vi "Setting_2.vi"() -> ()   [LabVIEW 2015]
uses:
  0.Control/Setting_Control_Main_Inspection_Item Action.ctl
  0.Control/Setting_Control_Main Action.ctl
  <vilib>/vision/Measure.llb/Edge Options.ctl
  <vilib>/vision/Measure.llb/Edge Polarity.ctl
  <vilib>/vision/Measure.llb/Straight Edge Options.ctl
  <vilib>/vision/Measure.llb/Straight Edge Process.ctl
  <vilib>/Utility/miscctls.llb/LVPointTypeDef.ctl
  0.Control/Setting_Control_Pattern Paremeter.ctl
  <vilib>/userdefined/High Color/IMAQdx.ctl
  <vilib>/vision/NI_Vision_Development_Module.lvlib
panel:
  in  "ROIsize":cluster{"Width":dbl, "Height":dbl}[](array[cluster])=[{"Width"=0.375, "Height"=0.2}, {"Width"=0.375, "Height"=0.2}, {"Width"=0.375, "Height"=0.2}, {"Width"=0.375, "Height"=0.2}]
  in  "Don't need to press Ctrl To ZoomIn/ZoomOut":bool
  in  "ROI數量":i32=4
  in  "檢測項目":T1
  in  "確認檢測項目":bool
  in  "Tab Control":enum32{"設定", "тX把计", "тY把计", "補正參數"}(tab)
  in  "單步測試":bool
  in  "連續測試":bool
  in  "取像":bool
  in  "連續取像":bool
  in  "離開":bool
  in  "匯入圖片":bool
  out "Coordinate System":T2 {"Measurement System"."Axis Reference" items=["Direct", "Indirect"]; "Measurement System"."Angle (deg)" format="%.2f"; "Measurement System"."Origin"."Y" format="%.2f"; "Measurement System"."Origin"."X" format="%.2f"; "Reference System"."Axis Reference" items=["Direct", "Indirect"]; "Reference System"."Angle (deg)" format="%.2f"; "Reference System"."Origin"."Y" format="%.2f"; "Reference System"."Origin"."X" format="%.2f"}
  in  "start path":path=path "D:/渦輪組裝機參數/Data 資料/Setting Data"
  in  "file (use dialog)":path=path "D:/渦輪組裝機參數/Data 資料/Setting Data"
  out "Main Axis 2":T3 {"Point2"."Y" format="%.2f"; "Point2"."X" format="%.2f"; "Point1"."Y" format="%.2f"; "Point1"."X" format="%.2f"}
  out "Secondary Axis 2":T3 {"Point2"."Y" format="%.2f"; "Point2"."X" format="%.2f"; "Point1"."Y" format="%.2f"; "Point1"."X" format="%.2f"}
  out "Main Axis":T3 {"Point2"."Y" format="%.2f"; "Point2"."X" format="%.2f"; "Point1"."Y" format="%.2f"; "Point1"."X" format="%.2f"}
  out "Secondary Axis":T3 {"Point2"."Y" format="%.2f"; "Point2"."X" format="%.2f"; "Point1"."Y" format="%.2f"; "Point1"."X" format="%.2f"}
  in  "Direction":u16(ring)
  in  "LayoutOptions":T4={"Show Search Area"=FALSE, "Show Search Lines"=FALSE, "Show Edges Found"=FALSE, "Show Result"=TRUE, "Search Area Color"=65280, "Search Lines Color"=255, "Edge Locations Color"=16776960, "Result Color"=16711680, "Overlay Group Name"=""}
  in  "Primary Line Fit Options":T5={"Number of Lines"=1, "Type"=enum."First Edge Rake", "Min. Score"=10.0, "Max. Score"=1000.0, "Orientation"=0.0, "Angle Range"=45.0, "Angle Tolerance"=1.0, "Step Size"=7, "Min. SNR (db)"=0.0, "Min. Points (%)"=25.0, "Hough Iterations"=5} {"Min. Points (%)" min=0.0 max=100.0; "Min. SNR (db)" min=0.0; "Max. Score" min=0.0 max=1024.0; "Min. Score" min=0.0 max=1024.0 step=1.0}
  in  "Secondary Line Fit Options":T5={"Number of Lines"=1, "Type"=enum."First Edge Rake", "Min. Score"=10.0, "Max. Score"=1000.0, "Orientation"=0.0, "Angle Range"=45.0, "Angle Tolerance"=1.0, "Step Size"=7, "Min. SNR (db)"=0.0, "Min. Points (%)"=25.0, "Hough Iterations"=5} {"Min. Points (%)" min=0.0 max=100.0; "Min. SNR (db)" min=0.0; "Max. Score" min=0.0 max=1024.0; "Min. Score" min=0.0 max=1024.0 step=1.0}
  in  "Options":T9={"Direction"=0, "Primary Edge Options"={"Edge Polarity"=0, "Kernel Size"=3, "Width"=3, "Minimum Edge Strength"=10.0, "Interpolation Type"=enum."Bilinear Fixed", "Data Processing Method"=enum."Average"}, "Secondary Edge Options"={"Edge Polarity"=0, "Kernel Size"=3, "Width"=3, "Minimum Edge Strength"=10.0, "Interpolation Type"=enum."Bilinear Fixed", "Data Processing Method"=enum."Average"}, "Show Search Area"=FALSE, "Show Search Lines"=FALSE, "Show Edges Found"=FALSE, "Show Result"=TRUE, "Search Area Color"=65280, "Search Lines Color"=255, "Edge Locations Color"=16776960, "Result Color"=16711680, "Overlay Group Name"=""} {"Secondary Edge Options"."Edge Polarity" items=["All Edges", "Rising Edges", "Falling Edges"]; "Secondary Edge Options"."Minimum Edge Strength" format="%.2f"; "Secondary Edge Options"."Width" step=2; "Secondary Edge Options"."Kernel Size" step=2; "Primary Edge Options"."Edge Polarity" items=["All Edges", "Rising Edges", "Falling Edges"]; "Primary Edge Options"."Minimum Edge Strength" format="%.2f"; "Primary Edge Options"."Width" step=2; "Primary Edge Options"."Kernel Size" step=2}
  out "Image":T10(plugin-control)
  out "Pattern":T10(plugin-control)
  out "Set action":T11
  in  "相機、光源":T12 {"光源亮度" step=1 scale=0.0..255.0; "相機選擇" items=["相機 1", "相機 2"]; "光源選擇" items=["光源 1", "光源 2"]}
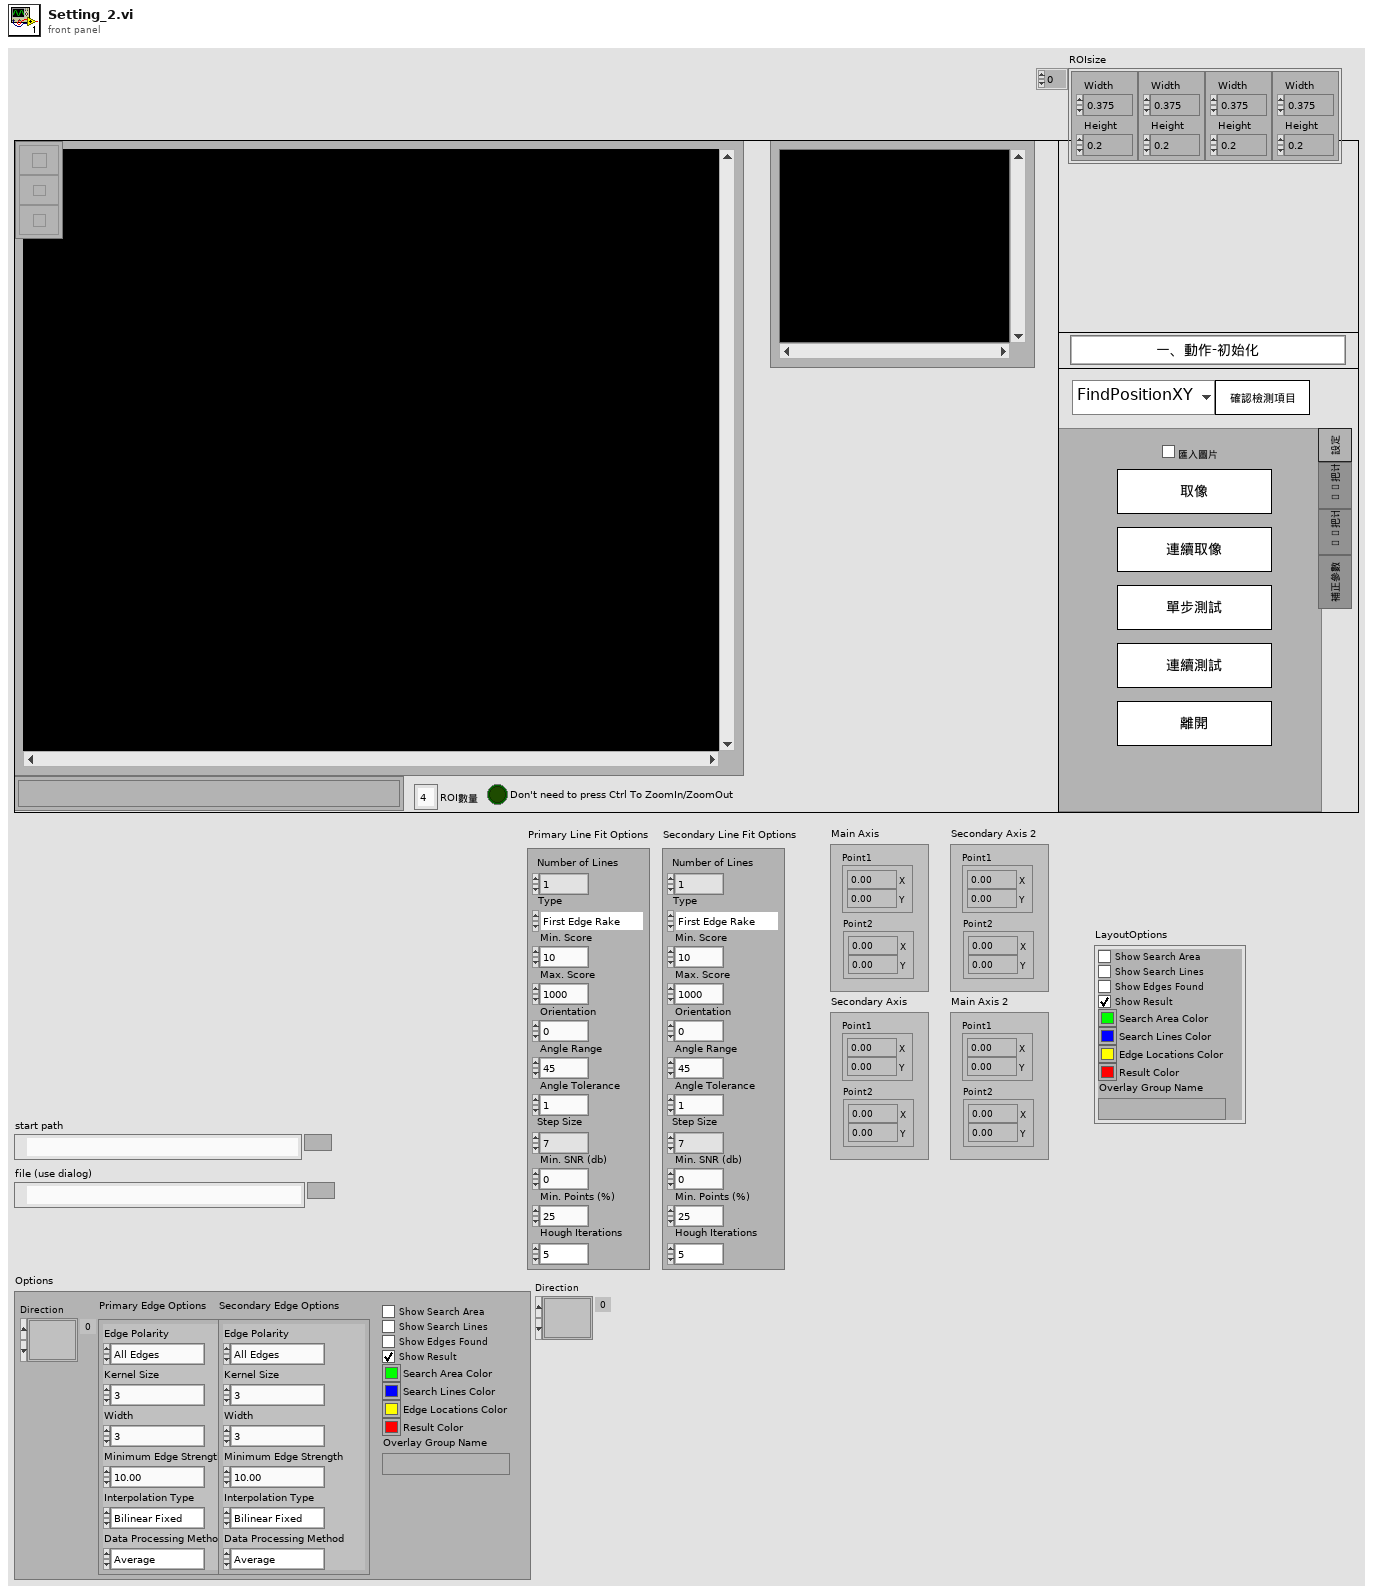
[diagram p1: front panel]
types:
  T1 = typedef "Setting_Control_Main_Inspection_Item Action.ctl" = enum16{"FindPositionXY", "Match"}
  T2 = typedef "IMAQ Coordinate System" = cluster{"Reference System":cluster{"Origin":cluster{"X":sgl, "Y":sgl}, "Angle (deg)":sgl, "Axis Reference":u32}, "Measurement System":cluster{"Origin":cluster{"X":sgl, "Y":sgl}, "Angle (deg)":sgl, "Axis Reference":u32}}
  T3 = cluster{"Point1":cluster{"X":sgl, "Y":sgl}, "Point2":cluster{"X":sgl, "Y":sgl}}
  T4 = cluster{"Show Search Area":bool, "Show Search Lines":bool, "Show Edges Found":bool, "Show Result":bool, "Search Area Color":u32, "Search Lines Color":u32, "Edge Locations Color":u32, "Result Color":u32, "Overlay Group Name":string}
  T5 = typedef "Straight Edge Options.ctl" = cluster{"Number of Lines":i32, "Type":T6, "Min. Score":dbl, "Max. Score":dbl, "Orientation":dbl, "Angle Range":dbl, "Angle Tolerance":dbl, "Step Size":u32, "Min. SNR (db)":dbl, "Min. Points (%)":dbl, "Hough Iterations":i32}
  T6 = typedef "Straight Edge Process.ctl" = enum32{"First Edge Rake", "Best Edge Rake", "Hough Edge Rake", "First Edge Projection", "Best Edge Projection"}
  T7 = typedef "Edge Options.ctl" = cluster{"Edge Polarity":T8, "Kernel Size":u32, "Width":u32, "Minimum Edge Strength":sgl, "Interpolation Type":enum32{"Zero Order", "Bilinear", "Quadratic", "Cubic", "Bilinear Fixed"}, "Data Processing Method":enum32{"Average", "Median"}}
  T8 = typedef "Edge Polarity.ctl" = u32
  T9 = cluster{"Direction":u16, "Primary Edge Options":T7, "Secondary Edge Options":T7, "Show Search Area":bool, "Show Search Lines":bool, "Show Edges Found":bool, "Show Result":bool, "Search Area Color":u32, "Search Lines Color":u32, "Edge Locations Color":u32, "Result Color":u32, "Overlay Group Name":string}
  T10 = typedef "IMAQ Image.ctl" = refnum<image>
  T11 = typedef "Setting_Control_Main Action.ctl" = enum16{"一、動作-初始化", "二、動作-單次取像", "三、動作-連續取像", "四、動作-單步測試", "五、動作-連續測試", "六、動作-離開", "1.0 功能-IO控制", "       1.1 IO-初始化", "       1.2 Set Point(EOT On)", "       1.3Set Point(EOT Off)", "       1.4Get Point(SOT)", "2.0功能-相機控制", "       2.1相機-初始化", "       2.2相機-取像", "       2.3相機-關閉", "3.0功能-影像控制", "       3.1影像-初始化", "       3.2影像-更新影像", "       3.3影像-儲存影像", "4.0功能-檢測", "       4.1檢測-初始化", "      4.2浪代-浪代", "             4.2.1浪代-FindEdgeX", "             4.2.2浪代-FindEdgeY", "             4.2.3浪代-FindPositionXY", "             4.2.4浪代-Match", "5.0功能-檔案", "       5.1檔案-初始化", "       5.2檔案-儲存檔案", "       5.3檔案-開啟檔案", "       5.4檔案-匯入檔案", "6.0 錯誤", "7.0等待", "       7.1等待(計算時間)", "8.0離開", "9.0功能-機台驗證", "      9.1機台驗證-初始化", "      9.2機台驗證-檢測", "10.0對話視窗", "11.光源控制", "       11.1光源控制-初始化", "       11.2光源控制-光源開啟", "       11.3光源控制-光源關閉", "       11.4光源控制-通訊關閉"}
  T12 = typedef "Control_Camera&Light.ctl" = cluster{"相機選擇":u8, "光源選擇":u16, "光源亮度":u8}
  T13 = typedef "LVPointTypeDef.ctl" = cluster{"Horizontal":i16, "Vertical":i16}
  T14 = typedef "光源通訊_action_control.ctl" = enum16{"initial", "開啟光源", "關閉光源", "close"}
  T15 = typedef "Control_Indicator Action(FGV).ctl" = enum16{"Set Data", "Get Data", "Idle"}
  T16 = typedef "Control_Indicator(FGV) #.ctl" = cluster{"相機、光源":cluster{"相機選擇":u8, "光源選擇":u16, "光源亮度":u8}, "Session Out":T17, "Cam#Light#Strength":string}
  T17 = typedef "IMAQdx.ctl" = refnum<k21>
  T18 = typedef "action_camera.ctl" = enum16{"初始化", "取像", "匯入影像", "結束"}
  T19 = typedef "Image action.ctl" = enum16{"初始化", "創造記憶體", "寫入圖片", "讀取圖片", "刪除圖片", "等待"}
  T20 = typedef "Setting_Control_Pattern Paremeter.ctl" = cluster{"方法":u16, "分數":sgl, "起始角度":sgl, "結束角度":sgl}
  T21 = cluster{"樣本比對參數L":T20, "ROI":cluster{"Global Rectangle":i32[], "Contours":cluster{"Contour Type":u32, "ROI Type":u32, "Points":i32[]}[]}, "Coordinate System Out":T2}
  T22 = typedef "Action_Data.ctl" = enum16{"Initialize", "Get Data", "Set Data", "Delete Data", "Idle"}
  T23 = cluster{"setting":cluster{"Contrast":i32, "Filter width":i32, "Steepness":i32, "Subsampling Ratio":u32}, "ROI":cluster{"Global Rectangle":i32[], "Contours":cluster{"Contour Type":u32, "ROI Type":u32, "Points":i32[]}[]}}
  T24 = cluster{"Scan Direction":u16, "ROI":cluster{"Global Rectangle":i32[], "Contours":cluster{"Contour Type":u32, "ROI Type":u32, "Points":i32[]}[]}, "Edge Options":T7}
  T25 = cluster{"Contrast":i32, "Filter width":i32, "Steepness":i32, "Subsampling Ratio":u32}
  T26 = typedef "Image Type" = u32
  T27 = cluster{"Global Rectangle":i32[], "Contours":cluster{"Contour Type":u32, "ROI Type":u32, "Points":i32[]}[]}
  T28 = cluster{"Position":cluster{"x":sgl, "y":sgl}, "Angle":sgl, "Scale":sgl, "Score":sgl, "Bounding Box":cluster{"x":sgl, "y":sgl}[]}[]
  T29 = cluster{"Position":cluster{"x":sgl, "y":sgl}, "Angle":sgl, "Scale":sgl, "Score":sgl, "Bounding Box":cluster{"x":sgl, "y":sgl}[]}
  T30 = typedef "ROI Descriptor" = cluster{"Global Rectangle":i32[], "Contours":cluster{"ID":enum32{"External", "Internal"}, "Type":u32, "Coordinates":i32[]}[]}
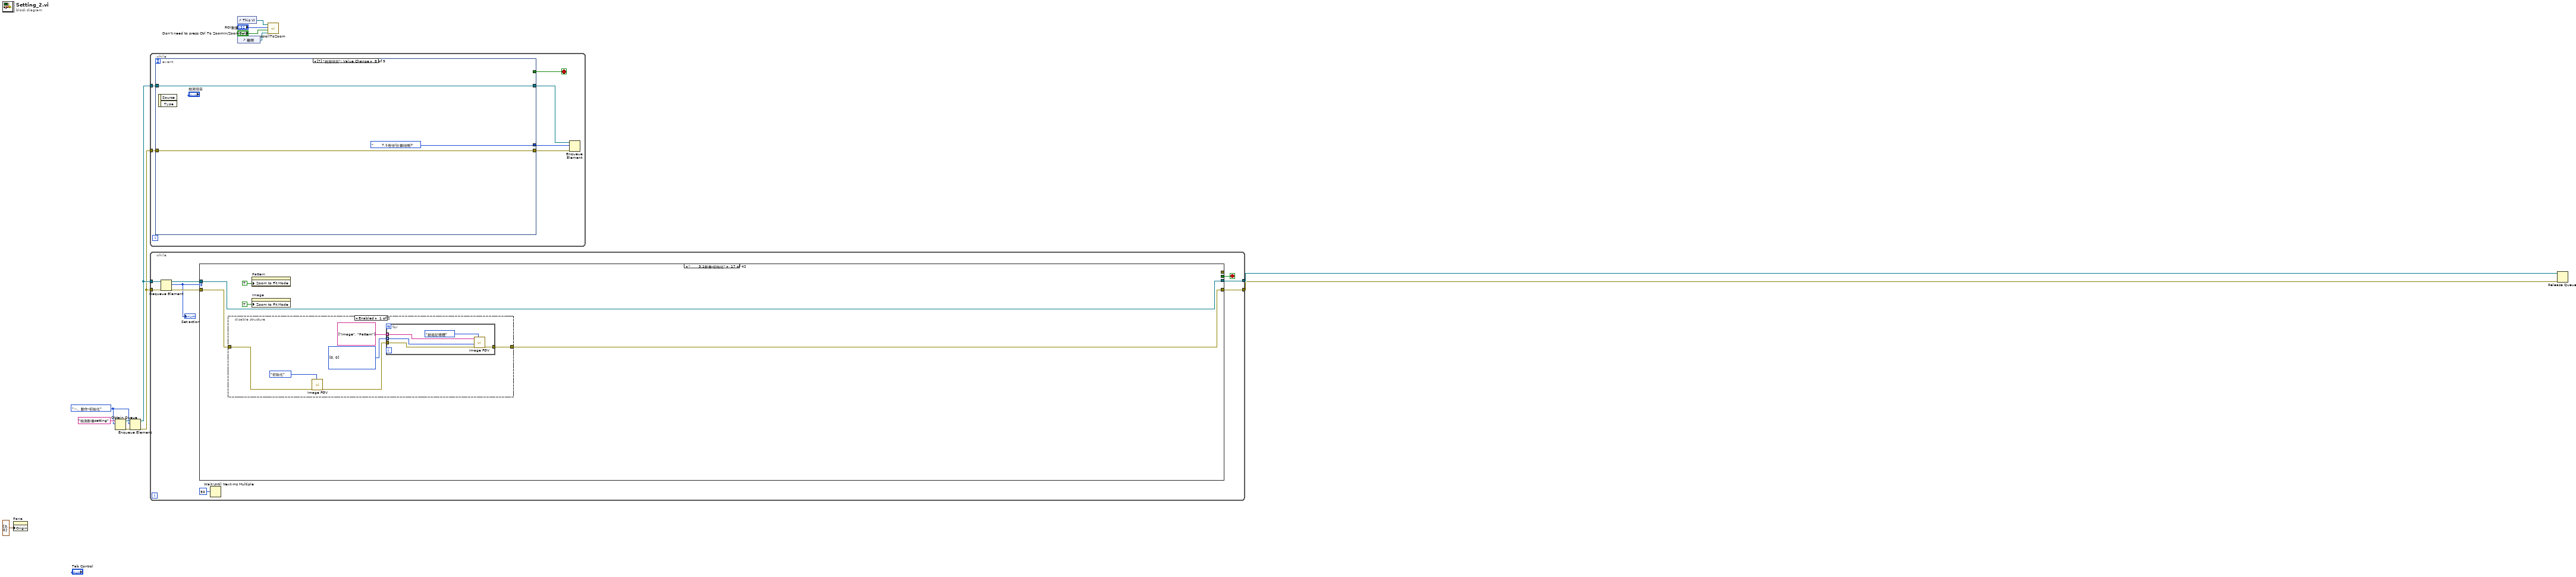
[diagram p0: block diagram]
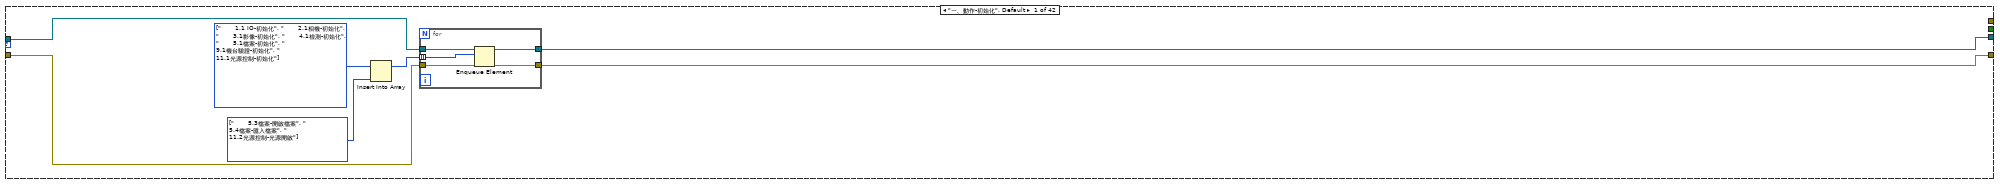
[diagram p2: hidden frame]
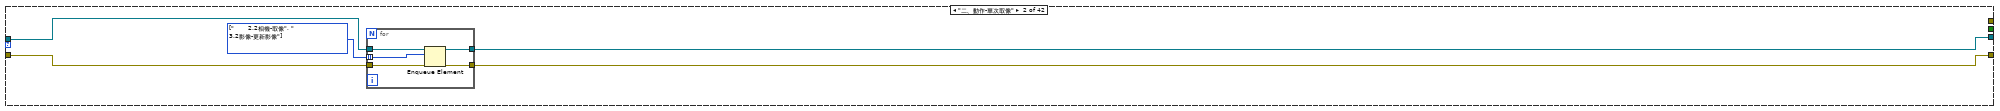
[diagram p3: hidden frame]
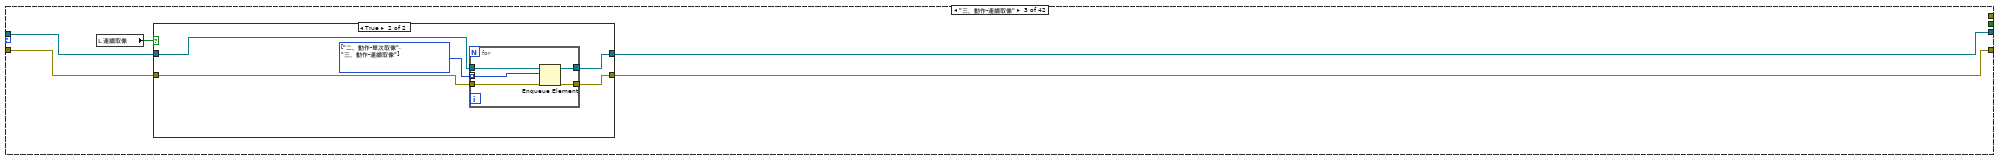
[diagram p4: hidden frame]
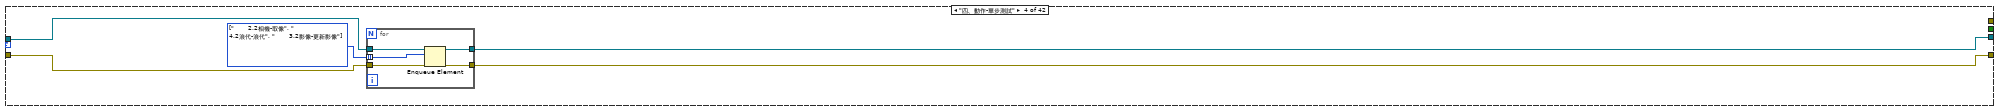
[diagram p6: hidden frame]
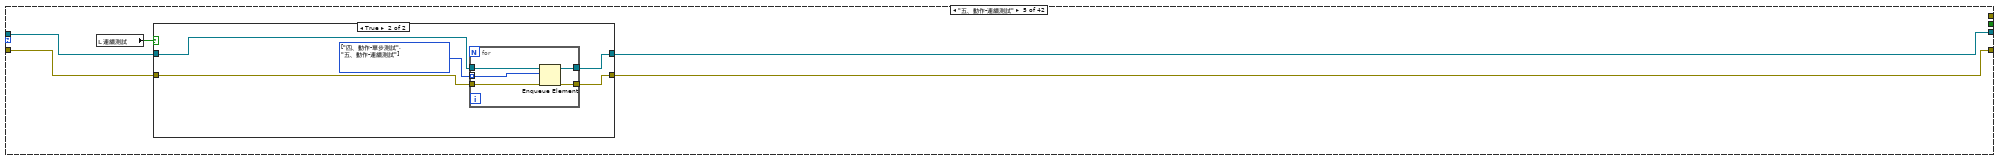
[diagram p7: hidden frame]
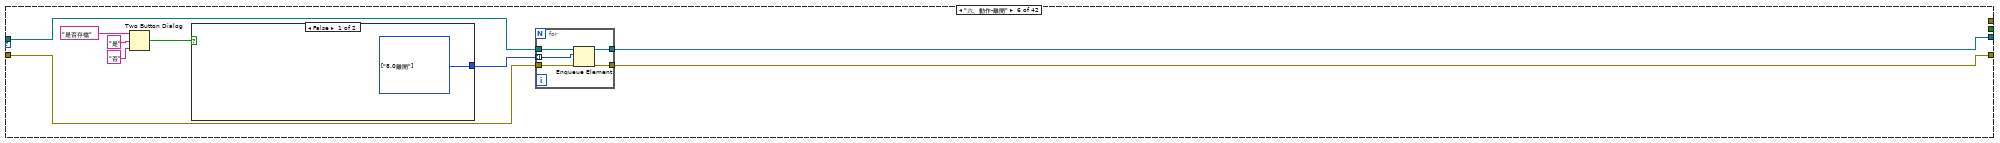
[diagram p9: hidden frame]
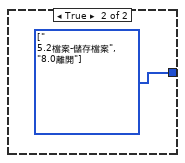
[diagram p10: hidden frame]
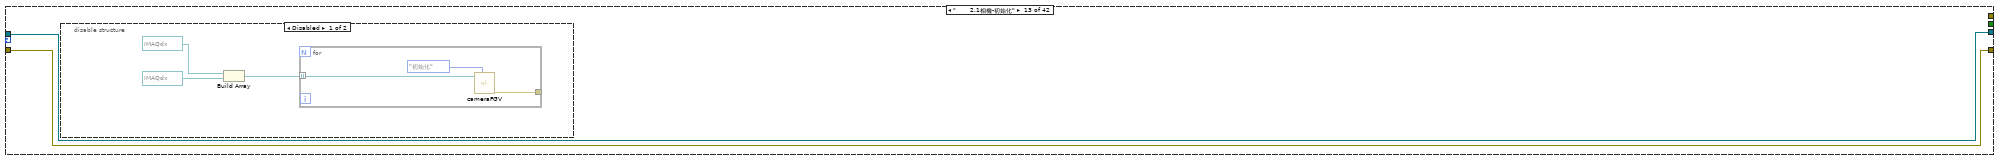
[diagram p17: hidden frame]
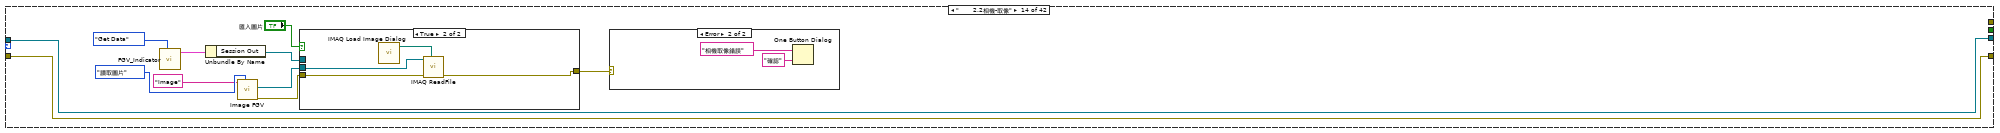
[diagram p19: hidden frame]
diagram:
  w1 = Setting_Control_Main_Action."一、動作-初始化" ("Set action")
  n1 = property on="Pane" class="Pane"("Origin"=T13 {"Horizontal"=0, "Vertical"=0}) -> ()  [unwired: 2 in, 2 out]
  n2 = Obtain Queue(name (unnamed)="檢測影像setting", element data type=w1) -> (queue out=w12:refnum<queue>, error out=w11:errorcluster)  [unwired: 3 in, 1 out]
  n3 = Enqueue Element(queue=w12, element=w1, error in (no error)=w11) -> (queue out=w10:refnum<queue>, error out=w9:errorcluster)  [unwired: 1 in, 1 out]
  n4 = while {
    tunnel: w10 -> [w19]
    tunnel: w9 -> [w18]
    stop <- w17 stop-if-true
    n5 = event shown="[7] \"檢測項目\": Value Change" {
      selector: _ -> [_ _ _ _ _ _ _ _ _]
      dyn-events: _ -> [_ _ _ _ _ _ _ _ _]
      timeout: _ -> [_ _ _ _ _ _ _ _ _]
      tunnel: w19 -> [w21 w24 w27 w30 w33 w36 w42 w52 w65]
      tunnel: [w21 w24 w27 w30 w33 w36 w41 w52 w65] -> w16
      tunnel: w18 -> [w20 w23 w26 w29 w32 w35 w40 w51 w64]
      tunnel: [w20 w23 w26 w29 w32 w35 w39 w51 w64] -> w15
      tunnel: [_ _ _ _ _ TRUE _ _ _] -> w17
      tunnel: [_ Setting_Control_Main_Action."二、動作-單次取像" ("Set action") Setting_Control_Main_Action."三、動作-連續取像" ("Set action") Setting_Control_Main_Action."四、動作-單步測試" ("Set action") Setting_Control_Main_Action."五、動作-連續測試" ("Set action") Setting_Control_Main_Action."六、動作-離開" ("Set action") w38 Setting_Control_Main_Action."       7.1等待(計算時間)" ("Set action") Setting_Control_Main_Action."       7.1等待(計算時間)" ("Set action")] -> w14
      event Timeout {
        n6 = event-data() -> ()  [unwired: 1 in, 3 out]
      }
      event "取像": Value Change {
        n7 = event-data() -> ()  [unwired: 1 in, 1 out]
      }
      event "連續取像": Value Change {
        n8 = event-data() -> ()  [unwired: 1 in, 1 out]
      }
      event "單步測試": Value Change {
        n9 = event-data() -> ()  [unwired: 1 in, 1 out]
      }
      event "連續測試": Value Change {
        n10 = event-data() -> ()  [unwired: 1 in, 1 out]
      }
      event "離開": Value Change {
        n11 = event-data() -> ()  [unwired: 1 in, 1 out]
      }
      event "確認檢測項目": Value Change {
        n12 = event-data() -> ()  [unwired: 1 in, 1 out]
        n13 = local read "檢測項目"() -> (w43:T1)
        n14 = case shown="\"Match\"" w43 {
          tunnel: w42 -> [w46 w49]
          tunnel: [w46 w49] -> w41
          tunnel: w40 -> [w45 w48]
          tunnel: [w45 w48] -> w39
          tunnel: [Setting_Control_Main_Action."             4.2.3浪代-FindPositionXY" ("Set action") Setting_Control_Main_Action."             4.2.4浪代-Match" ("Set action")] -> w38
          frame "FindPositionXY" {
          }
          frame "Match" {
          }
        }
      }
      event Value Change {
        n15 = event-data() -> ()  [unwired: 1 in, 2 out]
      }
      event Value Change {
        n16 = event-data() -> ()  [unwired: 1 in, 1 out]
        n17 = Bundle By Name(cluster=T16 {"相機、光源"={"相機選擇"=0, "光源選擇"=0, "光源亮度"=0}, "Session Out"="cam0", "Cam#Light#Strength"=""} ("Indicator Data In"), "相機、光源"="相機、光源") -> (w60:T16)
        n18 = Unbundle By Name("相機、光源") -> ("光源選擇"=w57:u16, "光源亮度"=w56:u8)  [unwired: 1 out]
        n19 = To Unsigned Byte Integer(number=w57) -> (unsigned 8bit integer=w55:u8)
        n20 = Increment(x=w55) -> (x+1=w54:u8)
        n21 = call "FGV_Indicator.vi"("Action"=Control_Indicator_Action(FGV)."Set Data", "Indicator Data In"=w60) -> ()  [unwired: 9 in, 1 out]
        n22 = call "光源通訊_FGV.vi"("通訊_action"=光源通訊_action_control."開啟光源", "亮度"=w56, "通道"=w54) -> ("error out"=w53:errorcluster)  [unwired: 7 in, 1 out]
        n23 = case shown="Error" w53 {
          frame No Error {
          }
          frame Error {
            n24 = One Button Dialog(message="光源開啟錯誤", button name ("OK")="確認") -> ()  [unwired: 1 out]
          }
        }
      }
    }
    n25 = Enqueue Element(queue=w16, element=w14, error in (no error)=w15) -> ()  [unwired: 1 in, 3 out]
  }
  n26 = while {
    tunnel: w10 -> [w76]
    tunnel: w9 -> [w75]
    tunnel: [w69] -> w8
    tunnel: [w70] -> w7
    stop <- w74 stop-if-true
    n27 = Dequeue Element(queue=w76, error in (no error)=w75) -> (queue out=w73:refnum<queue>, element=w68:T11, error out=w72:errorcluster)  [unwired: 1 in, 1 out]
    "Set action" <- w68
    n28 = case shown="\"       3.1影像-初始化\"" w68 {
      tunnel: [_ _ _ _ _ _ _ _ _ _ _ _ _ _ _ _ _ _ _ _ _ _ _ _ _ _ _ _ _ _ _ _ TRUE _ _ _ _ _ _ _ _ _] -> w74
      tunnel: w73 -> [w80 w93 w103 w120 w130 w151 w160 w162 w164 w166 w168 w170 w172 w185 w206 w214 w219 w242 w247 w249 w251 w262 w377 w467 w542 w545 w568 w587 w654 w667 w669 w671 w674 w676 w678 w680 w682 w684 w686 w700 w712 w716]
      tunnel: w72 -> [w83 w92 w102 w119 w129 w150 w159 w161 w163 w165 w167 w169 w171 w180 w205 w213 w217 w236 w246 w248 w250 w261 w380 w463 w541 w543 w567 w586 w653 w666 w668 w670 w673 w675 w677 w679 w681 w683 w685 w699 w711 w715]
      tunnel: [w81 w90 w101 w118 w128 w149 w160 w162 w164 w166 w168 w170 w172 w185 w206 w214 w219 w242 w247 w249 w251 w262 w384 w466 w542 w545 w568 w588 w654 w667 w669 w671 w674 w676 w678 w680 w682 w684 w686 w700 w712 w716] -> w69
      tunnel: [w82 w91 w100 w117 w127 w148 w159 w161 w163 w165 w167 w169 w171 w180 w205 w213 w216 w234 w246 w248 w250 w261 w378 w465 w541 w543 w567 w585 w653 w666 w668 w670 w673 w675 w677 w679 w681 w683 w685 w699 w711 w715] -> w70
      tunnel: [_ _ _ _ _ _ _ _ _ _ _ _ _ _ _ _ _ _ _ _ _ w260 _ _ _ _ _ w583 _ _ _ _ _ _ _ _ _ _ _ _ _ _] -> _
      frame "一、動作-初始化", Default {
        w77 = T11[] [enum."       5.3檔案-開啟檔案", enum."       5.4檔案-匯入檔案", enum."       11.2光源控制-光源開啟"] items=["一、動作-初始化", "二、動作-單次取像", "三、動作-連續取像", "四、動作-單步測試", "五、動作-連續測試", "六、動作-離開", "1.0 功能-IO控制", "       1.1 IO-初始化", "       1.2 Set Point(EOT On)", "       1.3Set Point(EOT Off)", "       1.4Get Point(SOT)", "2.0功能-相機控制", "       2.1相機-初始化", "       2.2相機-取像", "       2.3相機-關閉", "3.0功能-影像控制", "       3.1影像-初始化", "       3.2影像-更新影像", "       3.3影像-儲存影像", "4.0功能-檢測", "       4.1檢測-初始化", "      4.2浪代-浪代", "             4.2.1浪代-FindEdgeX", "             4.2.2浪代-FindEdgeY", "             4.2.3浪代-FindPositionXY", "             4.2.4浪代-Match", "5.0功能-檔案", "       5.1檔案-初始化", "       5.2檔案-儲存檔案", "       5.3檔案-開啟檔案", "       5.4檔案-匯入檔案", "6.0 錯誤", "7.0等待", "       7.1等待(計算時間)", "8.0離開", "9.0功能-機台驗證", "      9.1機台驗證-初始化", "      9.2機台驗證-檢測", "10.0對話視窗", "11.光源控制", "       11.1光源控制-初始化", "       11.2光源控制-光源開啟", "       11.3光源控制-光源關閉", "       11.4光源控制-通訊關閉"]
        w79 = T11[] [enum."       1.1 IO-初始化", enum."       2.1相機-初始化", enum."       3.1影像-初始化", enum."       4.1檢測-初始化", enum."       5.1檔案-初始化", enum."      9.1機台驗證-初始化", enum."       11.1光源控制-初始化"] items=["一、動作-初始化", "二、動作-單次取像", "三、動作-連續取像", "四、動作-單步測試", "五、動作-連續測試", "六、動作-離開", "1.0 功能-IO控制", "       1.1 IO-初始化", "       1.2 Set Point(EOT On)", "       1.3Set Point(EOT Off)", "       1.4Get Point(SOT)", "2.0功能-相機控制", "       2.1相機-初始化", "       2.2相機-取像", "       2.3相機-關閉", "3.0功能-影像控制", "       3.1影像-初始化", "       3.2影像-更新影像", "       3.3影像-儲存影像", "4.0功能-檢測", "       4.1檢測-初始化", "      4.2浪代-浪代", "             4.2.1浪代-FindEdgeX", "             4.2.2浪代-FindEdgeY", "             4.2.3浪代-FindPositionXY", "             4.2.4浪代-Match", "5.0功能-檔案", "       5.1檔案-初始化", "       5.2檔案-儲存檔案", "       5.3檔案-開啟檔案", "       5.4檔案-匯入檔案", "6.0 錯誤", "7.0等待", "       7.1等待(計算時間)", "8.0離開", "9.0功能-機台驗證", "      9.1機台驗證-初始化", "      9.2機台驗證-檢測", "10.0對話視窗", "11.光源控制", "       11.1光源控制-初始化", "       11.2光源控制-光源開啟", "       11.3光源控制-光源關閉", "       11.4光源控制-通訊關閉"]
        n29 = Insert Into Array(array=w79, new element=w77) -> (w78:T11[])  [unwired: 1 in]
        n30 = for {
          tunnel: w80 -> [w88]
          tunnel: w83 -> [w87]
          tunnel: [w86] -> w82
          tunnel: [w85] -> w81
          tunnel: w78 -> [w84] mode=indexing
          n31 = Enqueue Element(queue=w88, element=w84, error in (no error)=w87) -> (queue out=w85:refnum<queue>, error out=w86:errorcluster)  [unwired: 1 in, 1 out]
        }
      }
      frame "二、動作-單次取像" {
        w89 = T11[] [enum."       2.2相機-取像", enum."       3.2影像-更新影像"] items=["一、動作-初始化", "二、動作-單次取像", "三、動作-連續取像", "四、動作-單步測試", "五、動作-連續測試", "六、動作-離開", "1.0 功能-IO控制", "       1.1 IO-初始化", "       1.2 Set Point(EOT On)", "       1.3Set Point(EOT Off)", "       1.4Get Point(SOT)", "2.0功能-相機控制", "       2.1相機-初始化", "       2.2相機-取像", "       2.3相機-關閉", "3.0功能-影像控制", "       3.1影像-初始化", "       3.2影像-更新影像", "       3.3影像-儲存影像", "4.0功能-檢測", "       4.1檢測-初始化", "      4.2浪代-浪代", "             4.2.1浪代-FindEdgeX", "             4.2.2浪代-FindEdgeY", "             4.2.3浪代-FindPositionXY", "             4.2.4浪代-Match", "5.0功能-檔案", "       5.1檔案-初始化", "       5.2檔案-儲存檔案", "       5.3檔案-開啟檔案", "       5.4檔案-匯入檔案", "6.0 錯誤", "7.0等待", "       7.1等待(計算時間)", "8.0離開", "9.0功能-機台驗證", "      9.1機台驗證-初始化", "      9.2機台驗證-檢測", "10.0對話視窗", "11.光源控制", "       11.1光源控制-初始化", "       11.2光源控制-光源開啟", "       11.3光源控制-光源關閉", "       11.4光源控制-通訊關閉"]
        n32 = for {
          tunnel: w93 -> [w98]
          tunnel: w92 -> [w97]
          tunnel: [w96] -> w91
          tunnel: [w95] -> w90
          tunnel: w89 -> [w94] mode=indexing
          n33 = Enqueue Element(queue=w98, element=w94, error in (no error)=w97) -> (queue out=w95:refnum<queue>, error out=w96:errorcluster)  [unwired: 1 in, 1 out]
        }
      }
      frame "三、動作-連續取像" {
        n34 = local read "連續取像"() -> (w99:bool)
        n35 = case shown="True" w99 {
          tunnel: w103 -> [w105 w109]
          tunnel: w102 -> [w104 w108]
          tunnel: [w105 w107] -> w101
          tunnel: [w104 w106] -> w100
          frame False {
          }
          frame True {
            w110 = T11[] [enum."二、動作-單次取像", enum."三、動作-連續取像"] items=["一、動作-初始化", "二、動作-單次取像", "三、動作-連續取像", "四、動作-單步測試", "五、動作-連續測試", "六、動作-離開", "1.0 功能-IO控制", "       1.1 IO-初始化", "       1.2 Set Point(EOT On)", "       1.3Set Point(EOT Off)", "       1.4Get Point(SOT)", "2.0功能-相機控制", "       2.1相機-初始化", "       2.2相機-取像", "       2.3相機-關閉", "3.0功能-影像控制", "       3.1影像-初始化", "       3.2影像-更新影像", "       3.3影像-儲存影像", "4.0功能-檢測", "       4.1檢測-初始化", "      4.2浪代-浪代", "             4.2.1浪代-FindEdgeX", "             4.2.2浪代-FindEdgeY", "             4.2.3浪代-FindPositionXY", "             4.2.4浪代-Match", "5.0功能-檔案", "       5.1檔案-初始化", "       5.2檔案-儲存檔案", "       5.3檔案-開啟檔案", "       5.4檔案-匯入檔案", "6.0 錯誤", "7.0等待", "       7.1等待(計算時間)", "8.0離開", "9.0功能-機台驗證", "      9.1機台驗證-初始化", "      9.2機台驗證-檢測", "10.0對話視窗", "11.光源控制", "       11.1光源控制-初始化", "       11.2光源控制-光源開啟", "       11.3光源控制-光源關閉", "       11.4光源控制-通訊關閉"]
            n36 = for {
              tunnel: [w115] -> w106
              tunnel: [w114] -> w107
              tunnel: w110 -> [w113] mode=indexing
              tunnel: w109 -> [w112]
              tunnel: w108 -> [w111]
              n37 = Enqueue Element(queue=w112, element=w113, error in (no error)=w111) -> (queue out=w114:refnum<queue>, error out=w115:errorcluster)  [unwired: 1 in, 1 out]
            }
          }
        }
      }
      frame "四、動作-單步測試" {
        w116 = T11[] [enum."       2.2相機-取像", enum."      4.2浪代-浪代", enum."       3.2影像-更新影像"] items=["一、動作-初始化", "二、動作-單次取像", "三、動作-連續取像", "四、動作-單步測試", "五、動作-連續測試", "六、動作-離開", "1.0 功能-IO控制", "       1.1 IO-初始化", "       1.2 Set Point(EOT On)", "       1.3Set Point(EOT Off)", "       1.4Get Point(SOT)", "2.0功能-相機控制", "       2.1相機-初始化", "       2.2相機-取像", "       2.3相機-關閉", "3.0功能-影像控制", "       3.1影像-初始化", "       3.2影像-更新影像", "       3.3影像-儲存影像", "4.0功能-檢測", "       4.1檢測-初始化", "      4.2浪代-浪代", "             4.2.1浪代-FindEdgeX", "             4.2.2浪代-FindEdgeY", "             4.2.3浪代-FindPositionXY", "             4.2.4浪代-Match", "5.0功能-檔案", "       5.1檔案-初始化", "       5.2檔案-儲存檔案", "       5.3檔案-開啟檔案", "       5.4檔案-匯入檔案", "6.0 錯誤", "7.0等待", "       7.1等待(計算時間)", "8.0離開", "9.0功能-機台驗證", "      9.1機台驗證-初始化", "      9.2機台驗證-檢測", "10.0對話視窗", "11.光源控制", "       11.1光源控制-初始化", "       11.2光源控制-光源開啟", "       11.3光源控制-光源關閉", "       11.4光源控制-通訊關閉"]
        n38 = for {
          tunnel: w120 -> [w125]
          tunnel: w119 -> [w124]
          tunnel: [w123] -> w118
          tunnel: [w122] -> w117
          tunnel: w116 -> [w121] mode=indexing
          n39 = Enqueue Element(queue=w125, element=w121, error in (no error)=w124) -> (queue out=w123:refnum<queue>, error out=w122:errorcluster)  [unwired: 1 in, 1 out]
        }
      }
      frame "五、動作-連續測試" {
        n40 = local read "連續測試"() -> (w126:bool)
        n41 = case shown="True" w126 {
          tunnel: w130 -> [w132 w137]
          tunnel: w129 -> [w131 w136]
          tunnel: [w132 w135] -> w128
          tunnel: [w131 w134] -> w127
          frame False {
          }
          frame True {
            w133 = T11[] [enum."四、動作-單步測試", enum."五、動作-連續測試"] items=["一、動作-初始化", "二、動作-單次取像", "三、動作-連續取像", "四、動作-單步測試", "五、動作-連續測試", "六、動作-離開", "1.0 功能-IO控制", "       1.1 IO-初始化", "       1.2 Set Point(EOT On)", "       1.3Set Point(EOT Off)", "       1.4Get Point(SOT)", "2.0功能-相機控制", "       2.1相機-初始化", "       2.2相機-取像", "       2.3相機-關閉", "3.0功能-影像控制", "       3.1影像-初始化", "       3.2影像-更新影像", "       3.3影像-儲存影像", "4.0功能-檢測", "       4.1檢測-初始化", "      4.2浪代-浪代", "             4.2.1浪代-FindEdgeX", "             4.2.2浪代-FindEdgeY", "             4.2.3浪代-FindPositionXY", "             4.2.4浪代-Match", "5.0功能-檔案", "       5.1檔案-初始化", "       5.2檔案-儲存檔案", "       5.3檔案-開啟檔案", "       5.4檔案-匯入檔案", "6.0 錯誤", "7.0等待", "       7.1等待(計算時間)", "8.0離開", "9.0功能-機台驗證", "      9.1機台驗證-初始化", "      9.2機台驗證-檢測", "10.0對話視窗", "11.光源控制", "       11.1光源控制-初始化", "       11.2光源控制-光源開啟", "       11.3光源控制-光源關閉", "       11.4光源控制-通訊關閉"]
            n42 = for {
              tunnel: w137 -> [w142]
              tunnel: w136 -> [w141]
              tunnel: [w140] -> w135
              tunnel: [w139] -> w134
              tunnel: w133 -> [w138] mode=indexing
              n43 = Enqueue Element(queue=w142, element=w138, error in (no error)=w141) -> (queue out=w140:refnum<queue>, error out=w139:errorcluster)  [unwired: 1 in, 1 out]
            }
          }
        }
      }
      frame "六、動作-離開" {
        n44 = Two Button Dialog(message="是否存檔", 1:"否" ("F button name (\"Cancel\")"), 2:"是" ("T button name (\"OK\")")) -> (T button?=w147:bool)
        n45 = case shown="False" w147 {
          tunnel: [w152 w153] -> w143
          frame False {
            w152 = T11[] [enum."8.0離開"] items=["一、動作-初始化", "二、動作-單次取像", "三、動作-連續取像", "四、動作-單步測試", "五、動作-連續測試", "六、動作-離開", "1.0 功能-IO控制", "       1.1 IO-初始化", "       1.2 Set Point(EOT On)", "       1.3Set Point(EOT Off)", "       1.4Get Point(SOT)", "2.0功能-相機控制", "       2.1相機-初始化", "       2.2相機-取像", "       2.3相機-關閉", "3.0功能-影像控制", "       3.1影像-初始化", "       3.2影像-更新影像", "       3.3影像-儲存影像", "4.0功能-檢測", "       4.1檢測-初始化", "      4.2浪代-浪代", "             4.2.1浪代-FindEdgeX", "             4.2.2浪代-FindEdgeY", "             4.2.3浪代-FindPositionXY", "             4.2.4浪代-Match", "5.0功能-檔案", "       5.1檔案-初始化", "       5.2檔案-儲存檔案", "       5.3檔案-開啟檔案", "       5.4檔案-匯入檔案", "6.0 錯誤", "7.0等待", "       7.1等待(計算時間)", "8.0離開", "9.0功能-機台驗證", "      9.1機台驗證-初始化", "      9.2機台驗證-檢測", "10.0對話視窗", "11.光源控制", "       11.1光源控制-初始化", "       11.2光源控制-光源開啟", "       11.3光源控制-光源關閉", "       11.4光源控制-通訊關閉"]
          }
          frame True {
            w153 = T11[] [enum."       5.2檔案-儲存檔案", enum."8.0離開"] items=["一、動作-初始化", "二、動作-單次取像", "三、動作-連續取像", "四、動作-單步測試", "五、動作-連續測試", "六、動作-離開", "1.0 功能-IO控制", "       1.1 IO-初始化", "       1.2 Set Point(EOT On)", "       1.3Set Point(EOT Off)", "       1.4Get Point(SOT)", "2.0功能-相機控制", "       2.1相機-初始化", "       2.2相機-取像", "       2.3相機-關閉", "3.0功能-影像控制", "       3.1影像-初始化", "       3.2影像-更新影像", "       3.3影像-儲存影像", "4.0功能-檢測", "       4.1檢測-初始化", "      4.2浪代-浪代", "             4.2.1浪代-FindEdgeX", "             4.2.2浪代-FindEdgeY", "             4.2.3浪代-FindPositionXY", "             4.2.4浪代-Match", "5.0功能-檔案", "       5.1檔案-初始化", "       5.2檔案-儲存檔案", "       5.3檔案-開啟檔案", "       5.4檔案-匯入檔案", "6.0 錯誤", "7.0等待", "       7.1等待(計算時間)", "8.0離開", "9.0功能-機台驗證", "      9.1機台驗證-初始化", "      9.2機台驗證-檢測", "10.0對話視窗", "11.光源控制", "       11.1光源控制-初始化", "       11.2光源控制-光源開啟", "       11.3光源控制-光源關閉", "       11.4光源控制-通訊關閉"]
          }
        }
        n46 = for {
          tunnel: w151 -> [w158]
          tunnel: w150 -> [w157]
          tunnel: [w156] -> w149
          tunnel: [w155] -> w148
          tunnel: w143 -> [w154] mode=indexing
          n47 = Enqueue Element(queue=w158, element=w154, error in (no error)=w157) -> (queue out=w156:refnum<queue>, error out=w155:errorcluster)  [unwired: 1 in, 1 out]
        }
      }
      frame "1.0 功能-IO控制" {
      }
      frame "       1.1 IO-初始化" {
      }
      frame "       1.2 Set Point(EOT On)" {
      }
      frame "       1.3Set Point(EOT Off)" {
      }
      frame "       1.4Get Point(SOT)" {
      }
      frame "2.0功能-相機控制" {
      }
      frame "       2.1相機-初始化" {
        n48 = disable-structure shown="Disabled" {
          frame Disabled {
            n49 = Build Array(T17 "cam0" ("Session In"), T17 "cam1" ("Session In")) -> (w173:T17[])
            n50 = for {
              tunnel: w173 -> [w177] mode=indexing
              tunnel: [w176] -> _
              n51 = call "cameraFGV.vi"("action_camera"=action_camera."初始化", "Session In"=w177) -> ("error constant 2"=w176:errorcluster)  [unwired: 7 in, 2 out]
            }
          }
          frame Enabled {
          }
        }
      }
      frame "       2.2相機-取像" {
        n52 = call "FGV_Indicator.vi"("Action"=Control_Indicator_Action(FGV)."Get Data") -> ("Indicator Data Out"=w181:T16)  [unwired: 10 in]
        n53 = Unbundle By Name(w181) -> ("Session Out"=w183:T17)
        n54 = call "Image FGV.vi"("Image action"=Image_action."讀取圖片", "圖片名稱"="Image") -> ("error out"=w186:errorcluster, "Image Out"=w187:T10)  [unwired: 8 in]
        n55 = case shown="True" "匯入圖片" {
          tunnel: w187 -> [w200 w204]
          tunnel: w186 -> [w199 w203]
          tunnel: w183 -> [w195 _]
          tunnel: [w194 w201] -> w179
          frame False {
            n56 = call "cameraFGV.vi"("action_camera"=action_camera."取像", "error constant"=w199, "Image In"=w200, "Session In"=w195) -> ("error constant 2"=w198:errorcluster, "Image Out"=w197:T10)  [unwired: 5 in, 1 out]
            n57 = call "Image FGV.vi"("Image action"=Image_action."寫入圖片", "error in (no error)"=w198, "Image In"=w197, "圖片名稱"="Image") -> ("error out"=w194:errorcluster)  [unwired: 6 in, 1 out]
          }
          frame True {
            n58 = call "IMAQ Load Image Dialog"() -> ("Path"=w202:path)  [unwired: 9 in, 2 out]
            n59 = call "IMAQ ReadFile"("File Path"=w202, "error in (no error)"=w203, "Image"=w204) -> ("error out"=w201:errorcluster)  [unwired: 4 in, 4 out]
          }
        }
        n60 = case shown="Error" w179 {
          frame No Error {
          }
          frame Error {
            n61 = One Button Dialog(message="相機取像錯誤", button name ("OK")="確認") -> ()  [unwired: 1 out]
          }
        }
      }
      frame "       2.3相機-關閉" {
        n62 = disable-structure shown="Enabled" {
          frame Disabled {
            n63 = Build Array(T17 "cam0" ("Session In"), T17 "cam1" ("Session In")) -> (w207:T17[])
            n64 = for {
              tunnel: w207 -> [w211] mode=indexing
              tunnel: [w210] -> _
              n65 = call "cameraFGV.vi"("action_camera"=action_camera."結束", "Session In"=w211) -> ("error constant 2"=w210:errorcluster)  [unwired: 7 in, 2 out]
            }
          }
          frame Enabled {
          }
        }
      }
      frame "3.0功能-影像控制" {
      }
      frame "       3.1影像-初始化" {
        n66 = disable-structure shown="Enabled" {
          disable-tunnel: w217 -> [w221 w231]
          disable-tunnel: [w220 w231] -> w216
          frame Enabled {
            w222 = T26[] [0, 0] items=["Grayscale (U8)", "Grayscale (I16)", "Grayscale (SGL)", "Complex (CSG)", "RGB (U32)", "HSL (U32)", "RGB (U64)", "Grayscale (U16)"]
            n67 = call "Image FGV.vi"("Image action"=Image_action."初始化", "error in (no error)"=w221) -> ("error out"=w224:errorcluster)  [unwired: 8 in, 1 out]
            n68 = for {
              tunnel: w224 -> [w230]
              tunnel: string[] ["Image", "Pattern"] -> [w228] mode=indexing
              tunnel: w222 -> [w227] mode=indexing
              tunnel: [w226] -> w220
              n69 = call "Image FGV.vi"("Image action"=Image_action."創造記憶體", "error in (no error)"=w230, "Image Type"=w227, "圖片名稱"=w228) -> ("error out"=w226:errorcluster)  [unwired: 6 in, 1 out]
            }
          }
          frame Disabled {
          }
        }
        n70 = property on="Pattern" class="ImageControl"("Zoom to Fit Mode"=TRUE) -> ()  [unwired: 2 in, 2 out]
        n71 = property on="Image" class="ImageControl"("Zoom to Fit Mode"=TRUE) -> ()  [unwired: 2 in, 2 out]
      }
      frame "       3.2影像-更新影像" {
        n72 = call "Image FGV.vi"("Image action"=Image_action."讀取圖片", "error in (no error)"=w236, "圖片名稱"="Image") -> ("error out"=w235:errorcluster, "Image Out"=w233:T10)  [unwired: 7 in]
        n73 = disable-structure shown="Enabled" {
          disable-tunnel: w233 -> [w244 w245]
          disable-tunnel: [w243 w245] -> w232
          frame Disabled {
            n74 = call "點檢_VI_畫十字線.vi"("Refnum in"=w244) -> ("Refnum out"=w243:T10)  [unwired: 8 in, 2 out]
          }
          frame Enabled {
          }
        }
        "Image" <- w232
        n75 = call "Image FGV.vi"("Image action"=Image_action."讀取圖片", "error in (no error)"=w235, "圖片名稱"="Pattern") -> ("error out"=w234:errorcluster, "Image Out"=→"Pattern":T10)  [unwired: 7 in]
      }
      frame "       3.3影像-儲存影像" {
      }
      frame "4.0功能-檢測" {
      }
      frame "       4.1檢測-初始化" {
      }
      frame "      4.2浪代-浪代" {
        n76 = To Long Integer(number=Setting_Control_Main_Inspection_Item_Action."Match" ("檢測項目 2")) -> (32bit integer=w258:i32)
        n77 = call "FGV_Indicator.vi"("Action"=Control_Indicator_Action(FGV)."Get Data") -> ("Indicator Data Out"=w257:T16)  [unwired: 10 in]
        n78 = Unbundle By Name(w257) -> ("相機、光源"=w256:cluster{"相機選擇":u8, "光源選擇":u16, "光源亮度":u8})
        n79 = property on="檢測項目" class="Enum (strict)"() -> ("Strings []"=w259:string[])  [unwired: 2 in, 2 out]
        n80 = Unbundle By Name(w256) -> ("相機選擇"=w253:u8)
        n81 = Index Array(array=w259, index=w258) -> (element=w254:string)
        n82 = case shown="1" w253 {
          tunnel: w253 -> [w271 w341]
          tunnel: w254 -> [w270 w339]
          tunnel: [_ w296] -> w260
          tunnel: [w264 w293] -> _
          tunnel: [w263 w291] -> _
          frame 0, Default {
            w282 = u16 1 items=["Find Reference", "Update CoordSys"] ("Mode")
            n83 = Number To Decimal String(number=w271) -> (decimal integer string=w268:string)  [unwired: 1 in]
            n84 = Concatenate Strings(w270, "-" ("string"), w268) -> (w269:string)
            n85 = call "Main_FGV_Data.vi"("Action_Data"=Action_Data."Get Data", "Data name"=w269) -> ("Data  Out"=w279:cluster{"Data name":string, "Data":variant})  [unwired: 8 in, 1 out]
            n86 = Unbundle By Name(w279) -> ("Data"=w278:variant)
            n87 = Variant To Data(type=T21 {"樣本比對參數L"={"方法"=0, "分數"=0.0, "起始角度"=0.0, "結束角度"=0.0}, "ROI"={"Global Rectangle"=[], "Contours"=[]}, "Coordinate System Out"={"Reference System"={"Origin"={"X"=0.0, "Y"=0.0}, "Angle (deg)"=0.0, "Axis Reference"=0}, "Measurement System"={"Origin"={"X"=0.0, "Y"=0.0}, "Angle (deg)"=0.0, "Axis Reference"=0}}} ("output cluster"), Variant=w278) -> (data=w276:T21, error out=w266:errorcluster)  [unwired: 1 in]
            n88 = call "Image FGV.vi"("Image action"=Image_action."讀取圖片", "圖片名稱"="Image") -> ("Image Out"=w283:T10)  [unwired: 8 in, 1 out]
            n89 = call "Image FGV.vi"("Image action"=Image_action."讀取圖片", "圖片名稱"="Pattern") -> ("Image Out"=w281:T10)  [unwired: 8 in, 1 out]
            n90 = Unbundle(w276) -> ("樣本比對參數L"=w265:T20, "ROI"=w275:T27, "Coordinate System Out"=w274:T2)
            n91 = Unbundle By Name(w265) -> ("分數"=w263:sgl)
            n92 = call "浪代_Match_Sub.vi"("樣本比對參數"=w265, "ROI Descriptor"=w275, "Mode"=w282, "error in (no error)"=w266, "Coordinate System In"=w274, "Template Image"=w281, "Image"=w283) -> ("Matches (real-world)"=w273:T28)  [unwired: 1 in, 3 out]
            n93 = Index Array(array=w273) -> (element=w272:T29)  [unwired: 1 in]
            n94 = Unbundle By Name(w272) -> ("Score"=w264:sgl)  [unwired: 1 out]
          }
          frame 1 {
            w316 = u16 1 items=["Find Reference", "Update CoordSys"] ("Mode")
            n95 = disable-structure shown="Enabled" {
              disable-tunnel: ["找圓" ("string") "間距" ("element")] -> w335
              frame Disabled {
              }
              frame Enabled {
              }
            }
            n96 = Number To Decimal String(number=w341) -> (decimal integer string=w338:string)  [unwired: 1 in]
            n97 = Concatenate Strings(w339, "-" ("string"), w338) -> (w337:string)
            n98 = Build Array(w337, "找邊" ("string"), w335) -> (w332:string[])
            n99 = for {
              tunnel: w332 -> [w375] mode=indexing
              tunnel: [w374] -> w328 mode=indexing
              n100 = call "Main_FGV_Data.vi"("Action_Data"=Action_Data."Get Data", "Data name"=w375) -> ("Data  Out"=w374:cluster{"Data name":string, "Data":variant})  [unwired: 8 in, 1 out]
            }
            n101 = Index Array(array=w328, index #1=0 ("index"), index #2=1 ("index"), index #3=2 ("index")) -> (element #1=w327:cluster{"Data name":string, "Data":variant}, element #2=w326:cluster{"Data name":string, "Data":variant}, element #3=w325:cluster{"Data name":string, "Data":variant})
            n102 = Unbundle By Name(w327) -> ("Data"=w334:variant)
            n103 = Unbundle By Name(w326) -> ("Data"=w324:variant)
            n104 = Unbundle By Name(w325) -> ("Data"=w323:variant)
            n105 = Variant To Data(type=T21 {"樣本比對參數L"={"方法"=0, "分數"=0.0, "起始角度"=0.0, "結束角度"=0.0}, "ROI"={"Global Rectangle"=[], "Contours"=[]}, "Coordinate System Out"={"Reference System"={"Origin"={"X"=0.0, "Y"=0.0}, "Angle (deg)"=0.0, "Axis Reference"=0}, "Measurement System"={"Origin"={"X"=0.0, "Y"=0.0}, "Angle (deg)"=0.0, "Axis Reference"=0}}} ("output cluster"), Variant=w334) -> (data=w313:T21, error out=w308:errorcluster)  [unwired: 1 in]
            n106 = Variant To Data(type=T24 {"Scan Direction"=0, "ROI"={"Global Rectangle"=[], "Contours"=[]}, "Edge Options"={"Edge Polarity"=0, "Kernel Size"=0, "Width"=0, "Minimum Edge Strength"=0.0, "Interpolation Type"=enum."Zero Order", "Data Processing Method"=enum."Average"}} ("output cluster"), Variant=w324) -> (data=w304:T24, error out=w307:errorcluster)  [unwired: 1 in]
            n107 = Variant To Data(type=T23 {"setting"={"Contrast"=0, "Filter width"=0, "Steepness"=0, "Subsampling Ratio"=0}, "ROI"={"Global Rectangle"=[], "Contours"=[]}} ("output cluster"), Variant=w323) -> (data=w303:T23, error out=w306:errorcluster)  [unwired: 1 in]
            n108 = Merge Errors(w308, w307, w306) -> (w305:errorcluster)
            n109 = call "Image FGV.vi"("Image action"=Image_action."讀取圖片", "圖片名稱"="Pattern") -> ("Image Out"=w321:T10)  [unwired: 8 in, 1 out]
            n110 = call "Image FGV.vi"("Image action"=Image_action."讀取圖片", "圖片名稱"="Image") -> ("Image Out"=w298:T10)  [unwired: 8 in, 1 out]
            n111 = Unbundle(w313) -> ("樣本比對參數L"=w292:T20, "ROI"=w312:T27, "Coordinate System Out"=w311:T2)
            n112 = Unbundle By Name(w292) -> ("分數"=w291:sgl)
            n113 = call "浪代_Match_Sub.vi"("樣本比對參數"=w292, "ROI Descriptor"=w312, "Mode"=w316, "error in (no error)"=w305, "Coordinate System In"=w311, "Template Image"=w321, "Image"=w298) -> ("error out"=w310:errorcluster, "Coordinate System Out"=w302:T2, "Matches (real-world)"=w315:T28)  [unwired: 1 in, 1 out]
            n114 = Unbundle(w304) -> ("Scan Direction"=w301:u16, "ROI"=w300:T27, "Edge Options"=w299:T7)
            n115 = call "檢測_找邊_VI.vi"("Edge Options"=w299, "Scan Direction"=w301, "error in (no error)"=w310, "Coordinate System"=w302, "ROI"=w300, "Image"=w298) -> ("error out"=w309:errorcluster, "Array"=w295:cluster{"X":sgl, "Y":sgl}[])  [unwired: 3 in, 1 out]
            n116 = Index Array(array=w315) -> (element=w314:T29)  [unwired: 1 in]
            n117 = Unbundle By Name(w314) -> ("Score"=w293:sgl)  [unwired: 1 out]
            n118 = disable-structure shown="Enabled" {
              disable-tunnel: w309 -> [w364 w367]
              disable-tunnel: w303 -> [w363 w371]
              disable-tunnel: w302 -> [w362 w369]
              disable-tunnel: w298 -> [w358 w370]
              disable-tunnel: [w357 w366] -> w297
              disable-tunnel: [w356 _] -> w294
              disable-tunnel: [_ w365] -> w289
              frame Disabled {
                n119 = Unbundle(w363) -> (w361:T25, w360:T27, w359)
                n120 = call "檢測_找圓_VI.vi"("Edge Options"=w359, "Scan Direction"=w361, "error in (no error)"=w364, "Coordinate System"=w362, "ROI"=w360, "Image"=w358) -> ("error out"=w357:errorcluster, "Array"=w356:cluster{"X":sgl, "Y":sgl}[])  [unwired: 3 in, 1 out]
              }
              frame Enabled {
                n121 = Unbundle(w371) -> ("ROI"=w368:T27)  [unwired: 1 out]
                n122 = call "檢測_距離clamp_VI.vi"("error in (no error)"=w367, "Coordinate System"=w369, "ROI Descriptor"=w368, "Image"=w370) -> ("error out"=w366:errorcluster, "Distance"=w365:sgl)  [unwired: 4 in, 2 out]
              }
            }
            n123 = disable-structure shown="Enabled" {
              disable-tunnel: w298 -> [w346 w349]
              disable-tunnel: w297 -> [w345 _]
              disable-tunnel: [w344 _] -> w296
              disable-tunnel: w295 -> [w343 w351]
              disable-tunnel: w294 -> [w342 _]
              disable-tunnel: [_ w348] -> _
              disable-tunnel: [_ w347] -> w288
              frame Disabled {
                n124 = call "檢測_距離_VI.vi"("error in (no error)"=w345, "找圓"=w342, "找邊"=w343, "Image"=w346) -> ("error out"=w344:errorcluster)  [unwired: 4 in, 3 out]
              }
              frame Enabled {
                n125 = Index Array(array=w351) -> (element=w350:cluster{"X":sgl, "Y":sgl})  [unwired: 1 in]
                n126 = call "檢測_影像中心到邊距離.vi"("End Point"=w350, "Image"=w349) -> ("Distances"=w355:sgl[])  [unwired: 7 in, 2 out]
                n127 = Index Array(array=w355) -> (element=w354:sgl)  [unwired: 1 in]
                n128 = Divide(x=33.0, y=2592.0) -> (x/y=w347:dbl)
                n129 = Multiply(x=w354, y=w347) -> (x*y=w348:dbl)
              }
            }
            n130 = Multiply(x=w289, y=w288) -> ()  [unwired: 1 out]
          }
        }
      }
      frame "             4.2.3浪代-FindPositionXY" {
        n131 = flat-sequence {
          tunnel: [w397] -> w382
          tunnel: [w398] -> w381
          tunnel: w380 -> [w399]
          tunnel: [w438] -> w379
          tunnel: w382 -> [w440]
          tunnel: w381 -> [w439]
          frame #0 {
            w405 = u16 0 items=["Find Reference", "Update CoordSys"] ("Mode")
            n132 = flat-sequence {
              tunnel: [w437] -> w406
              tunnel: [w425] -> w389
              frame #0 {
                n133 = local read "LayoutOptions"() -> (w427:T4)
                n134 = local read "Direction"() -> (w425:u16)
                n135 = local read "Options"() -> (w426:T9)
                n136 = Unbundle(w427) -> ("Show Search Area"=w436:bool, "Show Search Lines"=w435:bool, "Show Edges Found"=w434:bool, "Show Result"=w433:bool, "Search Area Color"=w432:u32, "Search Lines Color"=w431:u32, "Edge Locations Color"=w430:u32, "Result Color"=w429:u32, "Overlay Group Name"=w428:string)
                n137 = Bundle(cluster=w426, "Direction"=w425, "Show Search Area"=w436, "Show Search Lines"=w435, "Show Edges Found"=w434, "Show Result"=w433, "Search Area Color"=w432, "Search Lines Color"=w431, "Edge Locations Color"=w430, "Result Color"=w429, "Overlay Group Name"=w428) -> (w437:T9)  [unwired: 2 in]
              }
            }
            n138 = local read "ROIsize"() -> (w385:cluster{"Width":dbl, "Height":dbl}[])
            n139 = property on="Image" class="ImageControl"() -> ("ROI"=w392:T27)  [unwired: 2 in, 2 out]
            n140 = call "Separate 4ROI_new2.vi"("ROI Descriptor"=w392, "ROIsize"=w385) -> ("Left ROI"=w396:T30, "Top ROI"=w395:T30, "Right ROI"=w394:T30, "Bottom ROI"=w393:T30)  [unwired: 9 in, 1 out]
            n141 = local read "Secondary Line Fit Options"() -> (w408:T5)
            n142 = case shown="1" w389 {
              tunnel: w396 -> [w410 w412 w413 _ _ _ _ w423]
              tunnel: w395 -> [_ w411 w414 w416 w417 _ _ _]
              tunnel: w394 -> [_ _ _ w415 w418 w420 w421 _]
              tunnel: w393 -> [w409 _ _ _ _ w419 w422 w424]
              tunnel: [w410 w412 w414 w416 w418 w420 w422 w424] -> w391
              tunnel: [w409 w411 w413 w415 w417 w419 w421 w423] -> w390
              frame 0, Default {
              }
              frame 1 {
                # "Second"
              }
              frame 2 {
              }
              frame 3 {
              }
              frame 4 {
              }
              frame 5 {
              }
              frame 6 {
              }
              frame 7 {
              }
            }
            n143 = local read "Primary Line Fit Options"() -> (w407:T5)
            n144 = local read "Coordinate System"() -> (w402:T2)
            n145 = call "Image FGV.vi"("Image action"=Image_action."讀取圖片", "圖片名稱"="Image") -> ("error out"=w386:errorcluster, "Image Out"=w388:T10)  [unwired: 8 in]
            n146 = call "IMAQ Clear Overlay"("error in (no error)"=w386, "Image"=w388) -> ("Image Out"=w387:T10)  [unwired: 8 in, 1 out]
            n147 = call "IMAQ Find CoordSys (2 Rects) 2"("Image"=w387, "Options"=w406, "Mode"=w405, "Primary ROI Descriptor"=w391, "Secondary ROI Descriptor"=w390, "Coordinate System In"=w402, "error in (no error)"=w399, "Primary Line Fit Options"=w407, "Secondary Line Fit Options"=w408) -> ("Main Axis"=→"Main Axis":T3, "Secondary Axis"=→"Secondary Axis":T3, "Coordinate System Out"=w397:T2, "error out"=w398:errorcluster)  [unwired: 2 in, 1 out]
            n148 = local write "Coordinate System"(w397) -> ()
          }
          frame #1 {
            n149 = Bundle("Coordinate System Out"=w440) -> (w445:cluster{"Coordinate System Out":T2})  [unwired: 1 in]
            n150 = case shown="Error" w439 {
              selector: w439 -> [w456 w457]
              tunnel: [w456 w457] -> w438
              frame No Error {
              }
              frame Error {
                n151 = One Button Dialog(message="match錯誤", button name ("OK")="確認") -> ()  [unwired: 1 out]
              }
            }
            n152 = To Variant(anything=w445) -> (Variant=w446:variant)
            n153 = local read "檢測項目"() -> (w443:T1)
            n154 = call "FGV_Indicator.vi"("Action"=Control_Indicator_Action(FGV)."Get Data") -> ("Indicator Data Out"=w448:T16)  [unwired: 10 in]
            n155 = Unbundle By Name(w448) -> ("相機、光源"=w449:cluster{"相機選擇":u8, "光源選擇":u16, "光源亮度":u8})
            n156 = To Long Integer(number=w443) -> (32bit integer=w442:i32)
            n157 = Unbundle By Name(w449) -> ("相機選擇"=w450:u8)
            n158 = property on="檢測項目" class="Enum (strict)"() -> ("Strings []"=w441:string[])  [unwired: 2 in, 2 out]
            n159 = Index Array(array=w441, index=w442) -> (element=w451:string)
            n160 = Number To Decimal String(number=w450) -> (decimal integer string=w453:string)  [unwired: 1 in]
            n161 = Concatenate Strings(w451, "-" ("string"), w453) -> (w455:string)
            n162 = Bundle(w455, "Variant"=w446) -> (w454:cluster{string, "Variant":variant})  [unwired: 1 in]
            n163 = call "Main_FGV_Data.vi"("Action_Data"=Action_Data."Set Data", "Data In"=w454, "Data name"=w455) -> ()  [unwired: 7 in, 2 out]
          }
        }
        n164 = Enqueue Element(queue=w377, element=Setting_Control_Main_Action."       3.2影像-更新影像", error in (no error)=w379) -> (queue out=w384:refnum<queue>, error out=w378:errorcluster)  [unwired: 1 in, 1 out]
      }
      frame "             4.2.4浪代-Match" {
        n165 = flat-sequence {
          tunnel: [w479] -> w461
          tunnel: [w480] -> w460
          tunnel: w463 -> [w481]
          tunnel: [w519] -> w462
          tunnel: w461 -> [w521]
          tunnel: w460 -> [w520]
          frame #0 {
            w487 = u16 1 items=["Find Reference", "Update CoordSys"] ("Mode")
            n166 = flat-sequence {
              tunnel: [w518] -> w488
              tunnel: [w507] -> w471
              frame #0 {
                n167 = local read "LayoutOptions"() -> (w509:T4)
                n168 = local read "Direction"() -> (w507:u16)
                n169 = local read "Options"() -> (w508:T9)
                n170 = Unbundle(w509) -> ("Show Search Area"=w517:bool, "Show Search Lines"=w516:bool, "Show Edges Found"=w515:bool, "Show Result"=w514:bool, "Search Area Color"=w513:u32, "Search Lines Color"=w512:u32, "Edge Locations Color"=w511:u32, "Result Color"=w510:u32)  [unwired: 1 out]
                n171 = Bundle(cluster=w508, "Direction"=w507, "Show Search Area"=w517, "Show Search Lines"=w516, "Show Edges Found"=w515, "Show Result"=w514, "Search Area Color"=w513, "Search Lines Color"=w512, "Edge Locations Color"=w511, "Result Color"=w510) -> (w518:T9)  [unwired: 3 in]
              }
            }
            n172 = local read "ROIsize"() -> (w468:cluster{"Width":dbl, "Height":dbl}[])
            n173 = property on="Image" class="ImageControl"() -> ("ROI"=w474:T27)  [unwired: 2 in, 2 out]
            n174 = call "Separate 4ROI_new2.vi"("ROI Descriptor"=w474, "ROIsize"=w468) -> ("Left ROI"=w478:T30, "Top ROI"=w477:T30, "Right ROI"=w476:T30, "Bottom ROI"=w475:T30)  [unwired: 9 in, 1 out]
            n175 = local read "Secondary Line Fit Options"() -> (w490:T5)
            n176 = case shown="1" w471 {
              tunnel: w478 -> [w492 w494 w495 _ _ _ _ w505]
              tunnel: w477 -> [_ w493 w496 w498 w499 _ _ _]
              tunnel: w476 -> [_ _ _ w497 w500 w502 w503 _]
              tunnel: w475 -> [w491 _ _ _ _ w501 w504 w506]
              tunnel: [w492 w494 w496 w498 w500 w502 w504 w506] -> w473
              tunnel: [w491 w493 w495 w497 w499 w501 w503 w505] -> w472
              frame 0, Default {
              }
              frame 1 {
                # "Second"
              }
              frame 2 {
              }
              frame 3 {
              }
              frame 4 {
              }
              frame 5 {
              }
              frame 6 {
              }
              frame 7 {
              }
            }
            n177 = local read "Primary Line Fit Options"() -> (w489:T5)
            n178 = local read "Coordinate System"() -> (w484:T2)
            n179 = call "Image FGV.vi"("Image action"=Image_action."讀取圖片", "圖片名稱"="Image") -> ("Image Out"=w470:T10)  [unwired: 8 in, 1 out]
            n180 = call "IMAQ Clear Overlay"("Image"=w470) -> ("Image Out"=w469:T10)  [unwired: 9 in, 1 out]
            n181 = call "IMAQ Find CoordSys (2 Rects) 2"("Image"=w469, "Options"=w488, "Mode"=w487, "Primary ROI Descriptor"=w473, "Secondary ROI Descriptor"=w472, "Coordinate System In"=w484, "error in (no error)"=w481, "Primary Line Fit Options"=w489, "Secondary Line Fit Options"=w490) -> ("Main Axis"=→"Main Axis 2":T3, "Secondary Axis"=→"Secondary Axis 2":T3, "Coordinate System Out"=w479:T2, "error out"=w480:errorcluster)  [unwired: 2 in, 1 out]
            n182 = local write "Coordinate System"(w479) -> ()
          }
          frame #1 {
            n183 = Bundle("Coordinate System Out"=w521) -> (w526:cluster{"Coordinate System Out":T2})  [unwired: 1 in]
            n184 = case shown="Error" w520 {
              selector: w520 -> [w537 w538]
              tunnel: [w537 w538] -> w519
              frame No Error {
              }
              frame Error {
                n185 = One Button Dialog(message="match錯誤", button name ("OK")="確認") -> ()  [unwired: 1 out]
              }
            }
            n186 = To Variant(anything=w526) -> (Variant=w527:variant)
            n187 = local read "檢測項目"() -> (w524:T1)
            n188 = call "FGV_Indicator.vi"("Action"=Control_Indicator_Action(FGV)."Get Data") -> ("Indicator Data Out"=w529:T16)  [unwired: 10 in]
            n189 = Unbundle By Name(w529) -> ("相機、光源"=w530:cluster{"相機選擇":u8, "光源選擇":u16, "光源亮度":u8})
            n190 = To Long Integer(number=w524) -> (32bit integer=w523:i32)
            n191 = Unbundle By Name(w530) -> ("相機選擇"=w531:u8)
            n192 = property on="檢測項目" class="Enum (strict)"() -> ("Strings []"=w522:string[])  [unwired: 2 in, 2 out]
            n193 = Index Array(array=w522, index=w523) -> (element=w532:string)
            n194 = Number To Decimal String(number=w531) -> (decimal integer string=w534:string)  [unwired: 1 in]
            n195 = Concatenate Strings(w532, "-" ("string"), w534) -> (w536:string)
            n196 = Bundle(w536, "Variant"=w527) -> (w535:cluster{string, "Variant":variant})  [unwired: 1 in]
            n197 = call "Main_FGV_Data.vi"("Action_Data"=Action_Data."Set Data", "Data In"=w535, "Data name"=w536) -> ()  [unwired: 7 in, 2 out]
          }
        }
        n198 = Enqueue Element(queue=w467, element=Setting_Control_Main_Action."       3.2影像-更新影像", error in (no error)=w462) -> (queue out=w466:refnum<queue>, error out=w465:errorcluster)  [unwired: 1 in, 1 out]
      }
      frame "5.0功能-檔案" {
      }
      frame "       5.1檔案-初始化" {
        n199 = call "Main_FGV_Data.vi"("Action_Data"=Action_Data."Initialize") -> ()  [unwired: 9 in, 2 out]
      }
      frame "       5.2檔案-儲存檔案" {
        # "#儲存檔案\n看此資料夾裡是否有東西\n有的話就砍掉，沒有就直接儲存"
        n200 = call "FGV_Indicator.vi"("Action"=Control_Indicator_Action(FGV)."Get Data") -> ("Indicator Data Out"=w556:T16)  [unwired: 10 in]
        n201 = Unbundle By Name(w556) -> ("Cam#Light#Strength"=w547:string)
        n202 = Unbundle By Name(w556) -> ("相機、光源"=w555:cluster{"相機選擇":u8, "光源選擇":u16, "光源亮度":u8})
        n203 = Unbundle By Name(w555) -> ("相機選擇"=w554:u8)
        n204 = Concatenate Strings(w547, ".png" ("string")) -> (w557:string)
        n205 = case shown="1" w554 {
          tunnel: ["CCD1-塑膠" "CCD2-彈簧"] -> w552
          frame 0, Default {
          }
          frame 1 {
          }
        }
        n206 = Build Path(base path="file (use dialog)", name or relative path=w552) -> (appended path=w549:path)
        n207 = File/Directory Info(path=w549) -> (size=w551:i64)  [unwired: 1 in, 6 out]
        n208 = Equal To 0?(x=w551) -> (x = 0?=w550:bool)
        n209 = case shown="False" w550 {
          tunnel: w549 -> [w569 w574]
          tunnel: [w569 w574] -> w548
          frame False {
            n210 = List Folder(path=w569) -> (filenames=w570:string[])  [unwired: 3 in, 3 out]
            n211 = for {
              tunnel: w570 -> [w572] mode=indexing
              tunnel: w569 -> [w573]
              n212 = Build Path(base path=w573, name or relative path=w572) -> (appended path=w571:path)
              n213 = Delete(path (use dialog)=w571) -> ()  [unwired: 4 in, 3 out]
            }
          }
          frame True {
          }
        }
        n214 = Build Path(base path=w548, name or relative path=w557) -> (appended path=w560:path)
        n215 = Build Path(base path=w548, name or relative path=w547) -> (appended path=w564:path)
        n216 = call "Main_FGV_Data.vi"("Action_Data"=Action_Data."Idle") -> ("Data Array out"=w565:cluster{"Data name":string, "Data":variant}[])  [unwired: 9 in, 1 out]
        n217 = Write to Binary File(file (use dialog)=w564, data=w565) -> (error out=w561:errorcluster)  [unwired: 4 in, 2 out]
        n218 = call "Image FGV.vi"("Image action"=Image_action."讀取圖片", "圖片名稱"="Pattern") -> ("Image Out"=w562:T10)  [unwired: 8 in, 1 out]
        n219 = call "IMAQ Write Image And Vision Info File 2"("error in (no error)"=w561, "File Path"=w560, "Image"=w562) -> ()  [unwired: 7 in, 2 out]
      }
      frame "       5.3檔案-開啟檔案" {
        # "#開啟檔案\n錯誤表示沒有開檔，並\n強制設為CCD1取像\n沒有錯誤表示有開檔"
        n220 = Enqueue Element(queue=w587, element=Setting_Control_Main_Action."       3.2影像-更新影像", error in (no error)=w586) -> (queue out=w588:refnum<queue>, error out=w585:errorcluster)  [unwired: 1 in, 1 out]
        n221 = call "File Dialog"("start path"="start path") -> ("selected path"=w582:path, "error out"=w598:errorcluster)  [unwired: 11 in, 2 out]
        n222 = call "Main_FGV_Data.vi"("Action_Data"=Action_Data."Idle") -> ("Data Array out"=w596:cluster{"Data name":string, "Data":variant}[])  [unwired: 9 in, 1 out]
        n223 = Read from Binary File(5:w596, 8:w598, 11:w582) -> (0:w590:errorcluster, 2:w595:cluster{"Data name":string, "Data":variant}[])  [unwired: 3 in, 2 out]
        n224 = Strip Path(path=w582) -> (stripped path=w579:path, name=w581:string)
        n225 = for {
          tunnel: w595 -> [w609] mode=indexing
          tunnel: w590 -> [_]
          n226 = Unbundle(w609) -> ("Data name"=w610:string)  [unwired: 1 out]
          n227 = call "Main_FGV_Data.vi"("Action_Data"=Action_Data."Set Data", "Data In"=w609, "Data name"=w610) -> ()  [unwired: 7 in, 2 out]
        }
        n228 = case shown="No Error" w590 {
          tunnel: w582 -> [w599 _]
          frame No Error {
            n229 = Strip Path(path=w599) -> (name=w601:string)  [unwired: 1 out]
            n230 = call "SubVI_Cam&Li_String.vi"("Data String In"=w601) -> ("相機、光源"=w603:T12)  [unwired: 10 in]
            n231 = Bundle By Name(cluster=T16 {"相機、光源"={"相機選擇"=0, "光源選擇"=0, "光源亮度"=0}, "Session Out"="cam0", "Cam#Light#Strength"="CCD11126"} ("Indicator Data In"), "相機、光源"=w603) -> (w604:T16)
            n232 = call "FGV_Indicator.vi"("Action"=Control_Indicator_Action(FGV)."Set Data", "Indicator Data In"=w604) -> ()  [unwired: 9 in, 1 out]
          }
          frame Error {
            n233 = Bundle By Name(cluster=T16 {"相機、光源"={"相機選擇"=0, "光源選擇"=0, "光源亮度"=0}, "Session Out"="cam0", "Cam#Light#Strength"=""} ("Indicator Data In"), "相機、光源"=cluster{"相機選擇":u8, "光源選擇":u16, "光源亮度":u8} {"相機選擇"=0, "光源選擇"=0, "光源亮度"=0}) -> (w606:T16)
            n234 = call "FGV_Indicator.vi"("Action"=Control_Indicator_Action(FGV)."Set Data", "Indicator Data In"=w606) -> ()  [unwired: 9 in, 1 out]
          }
        }
        n235 = Concatenate Strings(w581, ".png" ("string")) -> (w578:string)
        n236 = call "Image FGV.vi"("Image action"=Image_action."讀取圖片", "error in (no error)"=w590, "圖片名稱"="Pattern") -> ("error out"=w589:errorcluster, "Image Out"=w591:T10)  [unwired: 7 in]
        n237 = Build Path(base path=w579, name or relative path=w578) -> (appended path=w577:path)
        n238 = call "IMAQ Read Image And Vision Info"("File Path"=w577, "error in (no error)"=w589, "Image"=w591) -> ("error out"=w583:errorcluster)  [unwired: 6 in, 2 out]
      }
      frame "       5.4檔案-匯入檔案" {
        # "#匯入檔案\n有錯誤表示沒有匯入檔案所以給常數\n沒錯誤表示有匯入檔案直接給儲存參數"
        n239 = call "FGV_Indicator.vi"("Action"=Control_Indicator_Action(FGV)."Get Data") -> ("Indicator Data Out"=w651:T16)  [unwired: 10 in]
        n240 = Unbundle By Name(w651) -> ("相機、光源"=w644:cluster{"相機選擇":u8, "光源選擇":u16, "光源亮度":u8})
        n241 = local write "相機、光源"(w644) -> ()
        n242 = Unbundle By Name(w644) -> ("相機選擇"=w631:u8)
        n243 = property on="檢測項目" class="Enum (strict)"() -> ("Strings []"=w632:string[])  [unwired: 2 in, 2 out]
        n244 = To Long Integer(number=enum16{"Pattern", "Match", "找邊", "間距"}."Match" ("檢測項目塑膠蓋")) -> (32bit integer=w648:i32)
        n245 = To Long Integer(number=enum16{"Pattern", "Match", "找邊", "間距"}."找邊" ("檢測項目塑膠蓋")) -> (32bit integer=w641:i32)
        n246 = To Long Integer(number=enum16{"Pattern", "Match", "找邊", "間距"}."間距" ("檢測項目塑膠蓋")) -> (32bit integer=w634:i32)
        n247 = Index Array(array=w632, index=w648) -> (element=w630:string)
        n248 = Index Array(array=w632, index=w641) -> (element=w628:string)
        n249 = Index Array(array=w632, index=w634) -> (element=w627:string)
        n250 = Number To Decimal String(number=w631) -> (decimal integer string=w643:string)  [unwired: 1 in]
        n251 = Concatenate Strings(w630, "-" ("string"), w643) -> (w629:string)
        n252 = Build Array(w629, w628, w627) -> (w626:string[])
        n253 = for {
          tunnel: w626 -> [w658] mode=indexing
          tunnel: [w657] -> w625 mode=indexing
          n254 = call "Main_FGV_Data.vi"("Action_Data"=Action_Data."Get Data", "Data name"=w658) -> ("Data  Out"=w657:cluster{"Data name":string, "Data":variant})  [unwired: 8 in, 1 out]
        }
        n255 = Index Array(array=w625, index #1=0 ("index"), index #2=1 ("index"), index #3=2 ("index")) -> (element #1=w621:cluster{"Data name":string, "Data":variant}, element #2=w620:cluster{"Data name":string, "Data":variant}, element #3=w619:cluster{"Data name":string, "Data":variant})
        n256 = Unbundle By Name(w621) -> ("Data"=w650:variant)
        n257 = Unbundle By Name(w620) -> ("Data"=w640:variant)
        n258 = Unbundle By Name(w619) -> ("Data"=w633:variant)
        n259 = Variant To Data(type=T24 {"Scan Direction"=0, "ROI"={"Global Rectangle"=[], "Contours"=[]}, "Edge Options"={"Edge Polarity"=0, "Kernel Size"=0, "Width"=0, "Minimum Edge Strength"=0.0, "Interpolation Type"=enum."Zero Order", "Data Processing Method"=enum."Average"}} ("output cluster"), Variant=w640) -> (data=w638:T24, error out=w637:errorcluster)  [unwired: 1 in]
        n260 = Variant To Data(type=T23 {"setting"={"Contrast"=0, "Filter width"=0, "Steepness"=0, "Subsampling Ratio"=0}, "ROI"={"Global Rectangle"=[], "Contours"=[]}} ("output cluster"), Variant=w633) -> (data=w613:T23, error out=w618:errorcluster)  [unwired: 1 in]
        n261 = Variant To Data(type=T21 {"樣本比對參數L"={"方法"=0, "分數"=0.0, "起始角度"=0.0, "結束角度"=0.0}, "ROI"={"Global Rectangle"=[], "Contours"=[]}, "Coordinate System Out"={"Reference System"={"Origin"={"X"=0.0, "Y"=0.0}, "Angle (deg)"=0.0, "Axis Reference"=0}, "Measurement System"={"Origin"={"X"=0.0, "Y"=0.0}, "Angle (deg)"=0.0, "Axis Reference"=0}}} ("output cluster"), Variant=w650) -> (data=w647:T21, error out=w646:errorcluster)  [unwired: 1 in]
        n262 = Unbundle By Name(w638) -> ("Scan Direction"=w636:u16, "Edge Options"=w635:T7)
        n263 = Unbundle By Name(w613) -> ("setting"=w612:T25)
        n264 = case shown="No Error" w637 {
          tunnel: [w661 u16 0 ("Scan Direction")] -> _
          tunnel: w636 -> [w661 _]
          tunnel: w635 -> [w660 _]
          tunnel: [w660 T7 {"Edge Polarity"=0, "Kernel Size"=3, "Width"=3, "Minimum Edge Strength"=10.0, "Interpolation Type"=enum."Bilinear Fixed", "Data Processing Method"=enum."Average"} ("Edge Options")] -> _
          frame No Error {
          }
          frame Error {
          }
        }
        n265 = case shown="Error" w618 {
          tunnel: w612 -> [w655 _]
          tunnel: [w655 T25 {"Contrast"=40, "Filter width"=4, "Steepness"=2, "Subsampling Ratio"=5} ("setting")] -> _
          frame No Error {
          }
          frame Error {
          }
        }
        n266 = Unbundle By Name(w647) -> ("樣本比對參數L"=w645:T20)
        n267 = case shown="No Error" w646 {
          tunnel: w645 -> [w664 _]
          tunnel: [w664 T20 {"方法"=1, "分數"=800.0, "起始角度"=-5.0, "結束角度"=5.0} ("樣本比對參數L")] -> _
          frame No Error {
          }
          frame Error {
          }
        }
      }
      frame "6.0 錯誤" {
      }
      frame "7.0等待" {
      }
      frame "       7.1等待(計算時間)" {
      }
      frame "8.0離開" {
      }
      frame "9.0功能-機台驗證" {
      }
      frame "      9.1機台驗證-初始化" {
      }
      frame "      9.2機台驗證-檢測" {
      }
      frame "10.0對話視窗" {
      }
      frame "11.光源控制" {
      }
      frame "       11.1光源控制-初始化" {
        n268 = disable-structure shown="Disabled" {
          frame Disabled {
            n269 = call "RS232 Device.vi"() -> ("error out"=w687:errorcluster, "COM"=w688:refnum<visa-resource-name>)  [unwired: 10 in]
            n270 = call "光源通訊_FGV.vi"("通訊_action"=光源通訊_action_control."initial", "error in (no error)"=w687, "VISA resource name"=w688) -> ()  [unwired: 7 in, 2 out]
          }
          frame Enabled {
          }
        }
      }
      frame "       11.2光源控制-光源開啟" {
        n271 = call "FGV_Indicator.vi"("Action"=Control_Indicator_Action(FGV)."Get Data") -> ("Indicator Data Out"=w696:T16)  [unwired: 10 in]
        n272 = Unbundle By Name(w696) -> ("相機、光源"=w695:cluster{"相機選擇":u8, "光源選擇":u16, "光源亮度":u8})
        n273 = Unbundle By Name(w695) -> ("光源選擇"=w693:u16, "光源亮度"=w694:u8)
        n274 = To Unsigned Byte Integer(number=w693) -> (unsigned 8bit integer=w692:u8)
        n275 = Increment(x=w692) -> (x+1=w691:u8)
        n276 = call "光源通訊_FGV.vi"("通訊_action"=光源通訊_action_control."開啟光源", "亮度"=w694, "通道"=w691) -> ("error out"=w690:errorcluster)  [unwired: 7 in, 1 out]
        n277 = case shown="Error" w690 {
          frame No Error {
          }
          frame Error {
            n278 = One Button Dialog(message="光源開啟錯誤", button name ("OK")="確認") -> ()  [unwired: 1 out]
          }
        }
      }
      frame "       11.3光源控制-光源關閉" {
        n279 = call "FGV_Indicator.vi"("Action"=Control_Indicator_Action(FGV)."Get Data") -> ("Indicator Data Out"=w708:T16)  [unwired: 10 in]
        n280 = Unbundle By Name(w708) -> ("相機、光源"=w707:cluster{"相機選擇":u8, "光源選擇":u16, "光源亮度":u8})
        n281 = Unbundle By Name(w707) -> ("光源選擇"=w706:u16)  [unwired: 1 out]
        n282 = To Unsigned Byte Integer(number=w706) -> (unsigned 8bit integer=w705:u8)
        n283 = Increment(x=w705) -> (x+1=w704:u8)
        n284 = call "光源通訊_FGV.vi"("通訊_action"=光源通訊_action_control."關閉光源", "通道"=w704) -> ("error out"=w703:errorcluster)  [unwired: 8 in, 1 out]
        n285 = case shown="Error" w703 {
          frame No Error {
          }
          frame Error {
            n286 = One Button Dialog(message="光源關閉錯誤", button name ("OK")="確認") -> ()  [unwired: 1 out]
          }
        }
      }
      frame "       11.4光源控制-通訊關閉" {
        n287 = disable-structure shown="Disabled" {
          frame Disabled {
            n288 = call "光源通訊_FGV.vi"("通訊_action"=光源通訊_action_control."initial") -> ()  [unwired: 9 in, 2 out]
          }
          frame Enabled {
          }
        }
      }
    }
    n289 = Wait Until Next ms Multiple(millisecond multiple=u32 50) -> ()  [unwired: 1 out]
  }
  n290 = control-ref of="This VI"() -> (w5:refnum<vi>)
  n291 = control-ref of="離開"() -> (w2:refnum<vi>)
  n292 = call "scrollToZoom.vi"("stop"=w2, "Don't need to press Ctrl To ZoomIn/ZoomOut"="Don't need to press Ctrl To ZoomIn/ZoomOut", "ROI數量"="ROI數量", "VI in"=w5) -> ()  [unwired: 8 in]
  n293 = Release Queue(queue=w8, error in (no error)=w7) -> ()  [unwired: 1 in, 3 out]
